vi "write driver inputs.vi"(0 "Jx":dbl, 2 "Jy":dbl, 3 "R":dbl, 8 "stack prefix":string, 9 "theta (rad)":dbl, 10 "Jr":dbl, 11 "theta (deg)":dbl) -> ()   [LabVIEW 2023]
uses:
  <vilib>/Rock Robotics/Network Tables/NT Write Number.vi
  Global odometry.vi
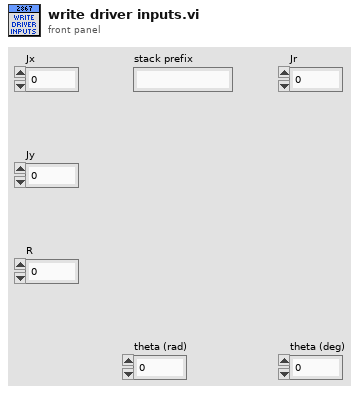
[diagram p1: front panel]
types:
  T1 = typedef "ctrl driver input.ctl" = cluster{"Jx":dbl, "Jy":dbl, "Jr ":dbl, "R":dbl, "theta (deg)":dbl, "theta (rad)":dbl, "DEADBAND?":bool, "FLD-CENTRIC?":bool, "HDG (deg)":dbl}
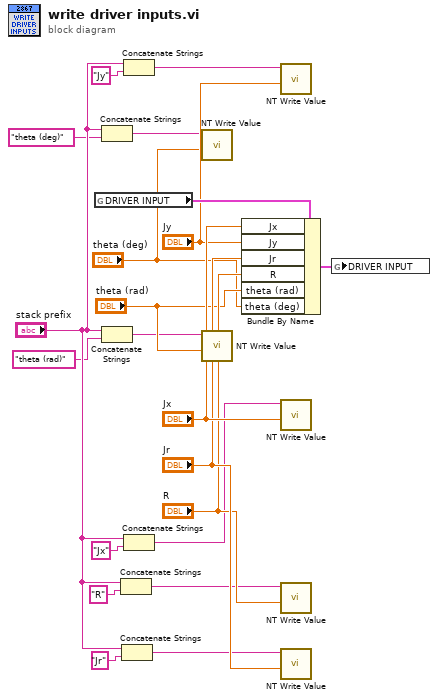
[diagram p0: block diagram]
diagram:
  n1 = global read "Global odometry.vi" "DRIVER INPUT"() -> (w21:T1)
  n2 = Concatenate Strings("stack prefix", "theta (deg)" ("string")) -> (w14:string)
  n3 = Concatenate Strings("stack prefix", "theta (rad)" ("string")) -> (w13:string)
  n4 = Concatenate Strings("stack prefix", "R" ("string")) -> (w12:string)
  n5 = Concatenate Strings("stack prefix", "Jr" ("string")) -> (w11:string)
  n6 = Concatenate Strings("stack prefix", "Jy" ("string")) -> (w10:string)
  n7 = Concatenate Strings("stack prefix", "Jx" ("string")) -> (w9:string)
  n8 = call-poly <vilib>:"NT Write Value.vi"("value"="theta (deg)", "name"=w14) -> ()  [unwired: 9 in, 1 out]
  n9 = call-poly <vilib>:"NT Write Value.vi"("value"="theta (rad)", "name"=w13) -> ()  [unwired: 9 in, 1 out]
  n10 = Bundle By Name(cluster=w21, "Jx"="Jx", "Jy"="Jy", "Jr"="Jr", "R"="R", "theta (rad)"="theta (rad)", "theta (deg)"="theta (deg)") -> (w1:T1)
  n11 = call-poly <vilib>:"NT Write Value.vi"("value"="Jy", "name"=w10) -> ()  [unwired: 9 in, 1 out]
  n12 = call-poly <vilib>:"NT Write Value.vi"("value"="Jx", "name"=w9) -> ()  [unwired: 9 in, 1 out]
  n13 = call-poly <vilib>:"NT Write Value.vi"("value"="R", "name"=w12) -> ()  [unwired: 9 in, 1 out]
  n14 = call-poly <vilib>:"NT Write Value.vi"("value"="Jr", "name"=w11) -> ()  [unwired: 9 in, 1 out]
  n15 = global write "Global odometry.vi" "DRIVER INPUT"(w1) -> ()
